vi "obj_DataLog Tag Hash.vi"(0 "method":T1=enum."index tag", 7 "tag in":string, 9 "tag index in":i32=-1, 11 "error in (no error)":errorcluster) -> (6 "#tags":i32, 8 "tag out":string, 10 "tag index out":i32, 15 "error out":errorcluster)   [LabVIEW 2012]
doc: "Efficiently associates the names of the tags in the live database with their indices. A tag index is required to access tag-specific data inside data structures set up for the live database. Only the {index tag}, {lookup}, and {#tags} methods are meant for public use. The {index tag} method retrieves the tag's name given a tag index. The {lookup} method retrieves the tag's index given a tag name. The {#tags} method returns the number of tags in the live database.\n\nBy storing the tag indices in a hash table, a lookup of a tag's index via its name becomes an O(1) operation (the execution time is independent of the number of tags). In this way, the amount of work during repeated run-time operations is reduced by proper preparation during the once-only initialization.\n\nNOTE: the subVIs for accessing the live database mostly accept both tag indices and tag names. In the latter case, they use this object to {lookup} the tag index."
uses:
  typedefs/t_DataLog Tag Hash Methods.ctl
  subvis/private/glb_DataLog Runtime Parameterisation.vi
  subvis/private/glb_DataLog MCVD.vi
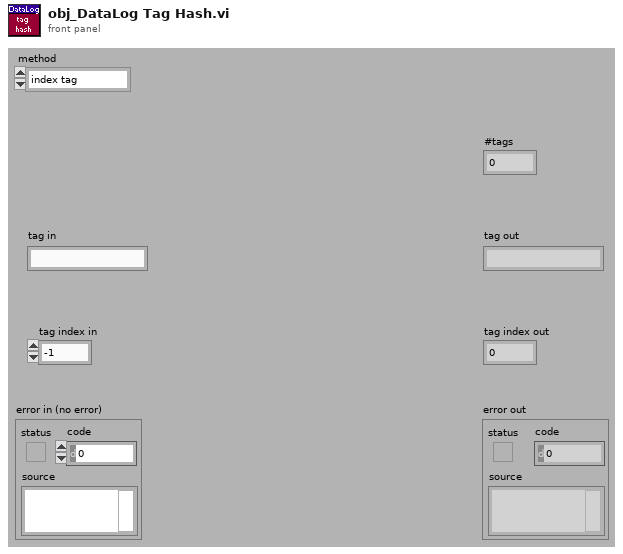
[diagram p1: front panel]
types:
  T1 = typedef "t_DataLog Tag Hash Methods.ctl" = enum16{"initialize", "add tag", "index tag", "lookup", "#tags", "cleanup", "write recovery", "read recovery", "delete recovery"}
  T2 = enum16{"deny read/write", "deny write-only", "deny none"}
  T3 = enum16{"read/write", "read-only", "write-only", "write-only (truncate)"}
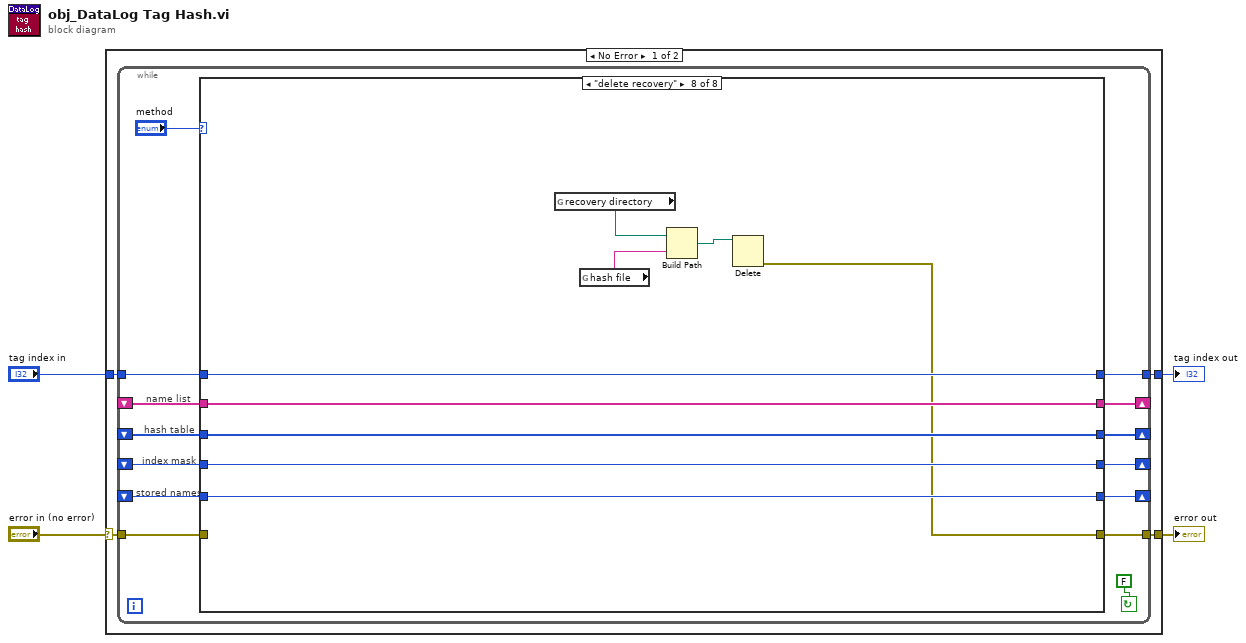
[diagram p0: block diagram]
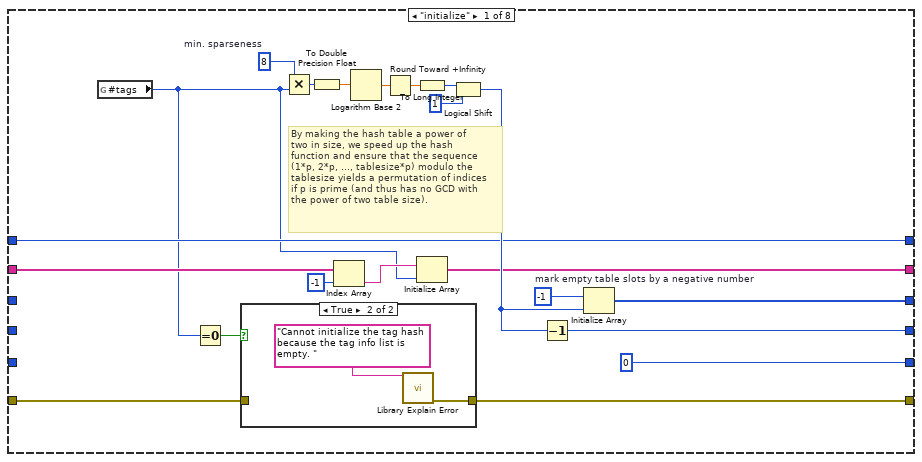
[diagram p2: hidden frame]
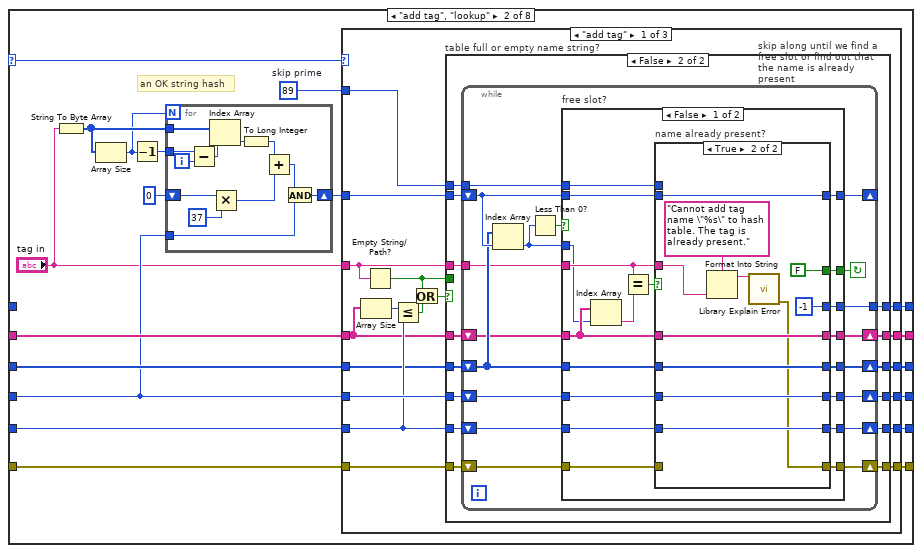
[diagram p4: hidden frame]
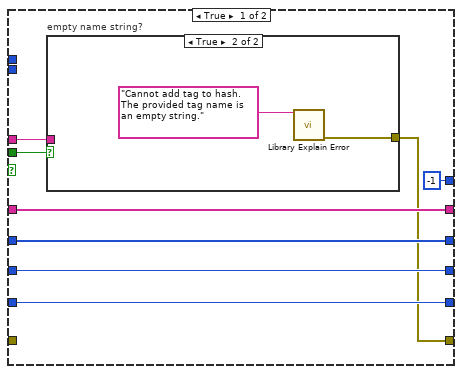
[diagram p5: hidden frame]
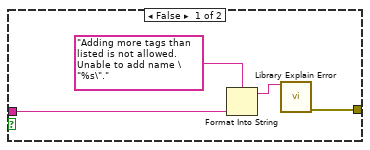
[diagram p6: hidden frame]
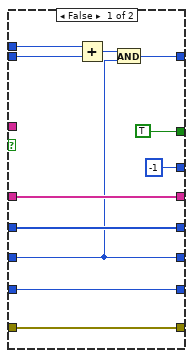
[diagram p7: hidden frame]
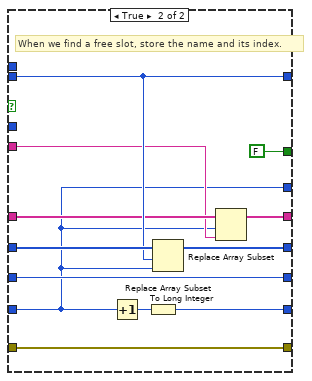
[diagram p8: hidden frame]
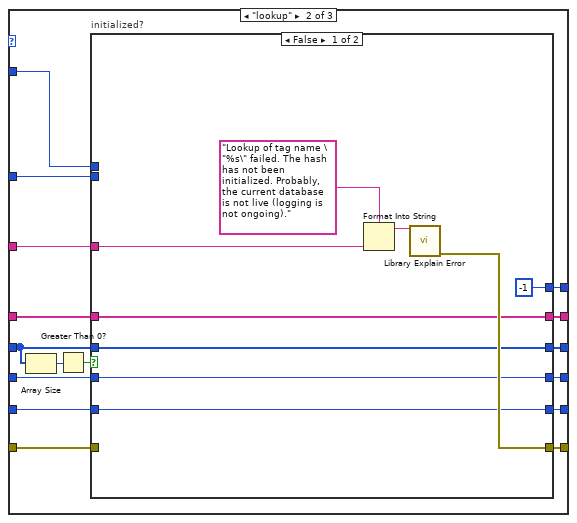
[diagram p9: hidden frame]
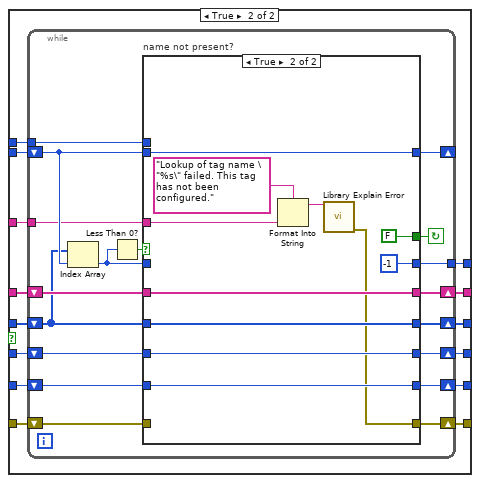
[diagram p10: hidden frame]
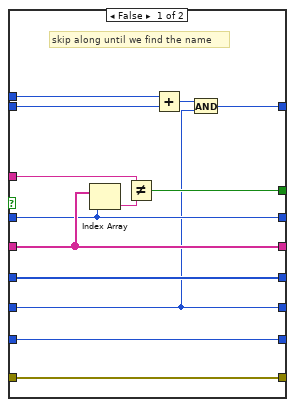
[diagram p11: hidden frame]
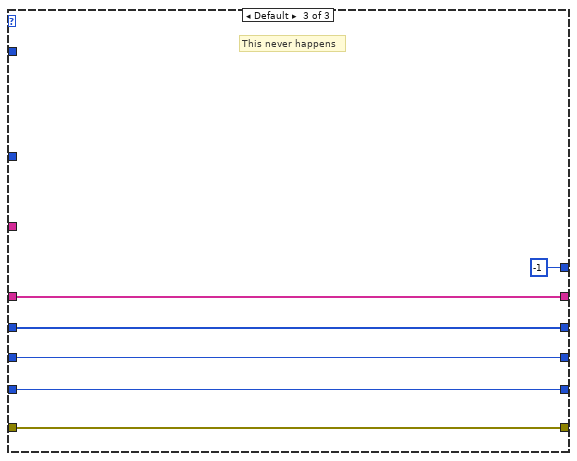
[diagram p12: hidden frame]
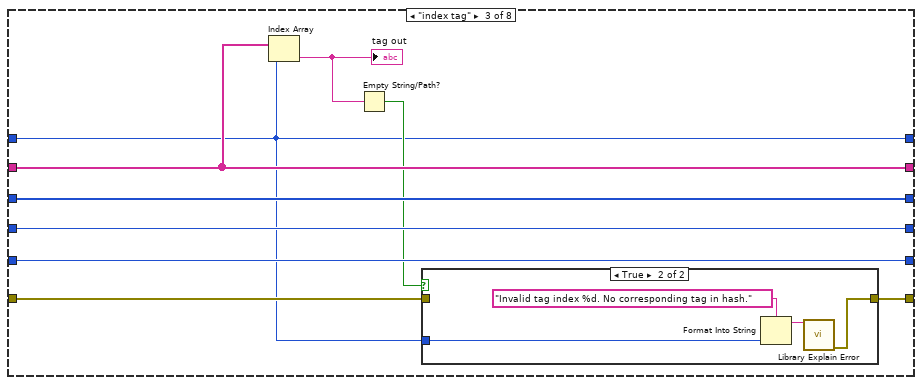
[diagram p13: hidden frame]
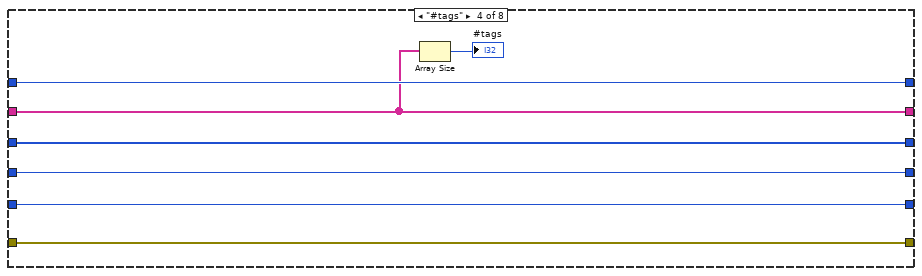
[diagram p15: hidden frame]
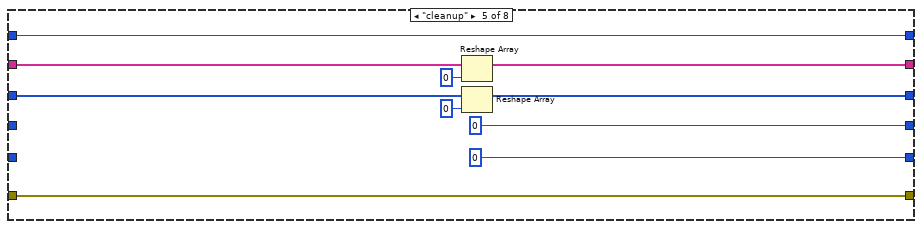
[diagram p16: hidden frame]
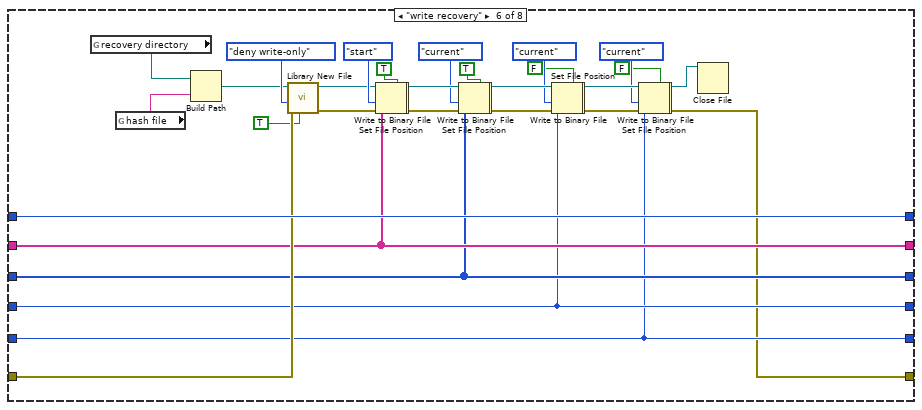
[diagram p17: hidden frame]
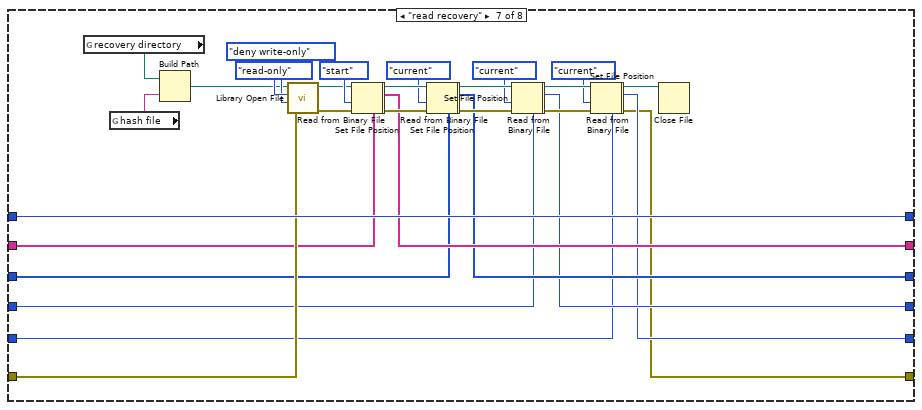
[diagram p18: hidden frame]
diagram:
  n1 = case shown="No Error" "error in (no error)" {
    selector: "error in (no error)" -> [w8 w397]
    tunnel: [w7 w397] -> w3
    tunnel: "tag index in" -> [w6 w396]
    tunnel: [w5 w396] -> w1
    frame No Error {
      n2 = while {
        shift-right: [w21] -> _
        shift-left: _ -> [w16]
        tunnel: w8 -> [w14]
        tunnel: [w20] -> w7
        shift-right: [w19] -> _
        shift-left: _ -> [w17]
        shift-right: [w18] -> _
        shift-left: _ -> [w15]
        tunnel: w6 -> [w12]
        tunnel: [w11] -> w5
        shift-right: [w9] -> _
        shift-left: _ -> [w10]
        stop <- FALSE continue-if-true
        # "stored names"
        # "index mask"
        # "name list"
        # "hash table"
        n3 = case shown="\"delete recovery\"" "method" {
          selector: "method" -> [_ w52 _ _ _ _ _ _]
          tunnel: w16 -> [_ w57 w289 w301 w306 w332 w366 w391]
          tunnel: [w31 w58 w289 w301 w305 w332 w367 w391] -> w21
          tunnel: w14 -> [w24 w53 w284 w299 w312 w334 w370 _]
          tunnel: [w26 w54 w283 w299 w312 w324 w359 w388] -> w20
          tunnel: w17 -> [w28 w60 w287 w297 w308 w333 w369 w392]
          tunnel: [w27 w59 w287 w297 w307 w333 w368 w392] -> w19
          tunnel: [w34 w55 w290 w302 0 w331 w365 w390] -> w18
          tunnel: w15 -> [_ w56 w290 w302 _ w331 w364 w390]
          tunnel: w12 -> [w32 _ w282 w298 w310 w349 w386 w395]
          tunnel: [w32 w61 w282 w298 w310 w349 w386 w395] -> w11
          tunnel: w10 -> [_ w49 w288 w300 _ w330 w362 w389]
          tunnel: [0 w48 w288 w300 0 w330 w363 w389] -> w9
          frame "initialize" {
            w36 = -1  # mark empty table slots by a negative number
            w37 = 8  # min. sparseness
            # "By making the hash table a power of\ntwo in size, we speed up the hash\nfunction and ensure that the sequence\n(1*p, 2*p, ..., tablesize*p) modulo the\ntablesize yields a permutation of indices\nif p is prime (and thus has no GCD with\nthe power of two table size)."
            n4 = global read "glb_DataLog Runtime Parameterisation.vi" "#tags"() -> (w23:i32)
            n5 = Equal To 0?(x=w23) -> (x = 0?=w25:bool)
            n6 = case shown="True" w25 {
              tunnel: [w44 w46] -> w26
              tunnel: w24 -> [w44 _]
              frame False {
              }
              frame True {
                n7 = call "Library Explain Error.vi"("explanation prefix (none)"="Cannot initialize the tag hash because the tag info list is empty. " ("explanation")) -> ("explained error"=w46:errorcluster)  [unwired: 14 in]
              }
            }
            n8 = Multiply(x=w37, y=w23) -> (x*y=w38:i32)
            n9 = To Double Precision Float(number=w38) -> (double precision float=w43:dbl)
            n10 = Index Array(array=w28, index=-1) -> (element=w29:string)
            n11 = Logarithm Base 2(1:w43) -> (0:w42:dbl)
            n12 = Round Toward +Infinity(x=w42) -> (ceil(x): smallest int >= x=w41:dbl)
            n13 = To Long Integer(number=w41) -> (32bit integer=w40:i32)
            n14 = Initialize Array(w29, w23) -> (w27:string[])
            n15 = Logical Shift(y=w40, x=1) -> (x << y=w35:i32)
            n16 = Decrement(x=w35) -> (x-1=w34:i32)
            n17 = Initialize Array(w36, w35) -> (w31:i32[])
          }
          frame "add tag", "lookup" {
            w47 = 89  # skip prime
            # "an OK string hash"
            n18 = String To Byte Array(string="tag in") -> (unsigned byte array=w64:u8[])
            n19 = Array Size(array=w64) -> (size(s)=w62:i32)
            n20 = Decrement(x=w62) -> (x-1=w63:i32)
            n21 = for {
              N: w62 -> [_]
              shift-right: [w275] -> w50
              shift-left: 0 -> [w276]
              tunnel: w64 -> [w279]
              tunnel: w63 -> [w281]
              tunnel: w56 -> [w274]
              i -> [w280]
              n22 = Subtract(x=w281, y=w280) -> (x-y=w278:i32)
              n23 = Index Array(array=w279, index=w278) -> (element=w273:u8)
              n24 = Multiply(x=w276, y=37 ("x")) -> (x*y=w272:i32)
              n25 = To Long Integer(number=w273) -> (32bit integer=w271:i32)
              n26 = Add(x=w271, y=w272) -> (x+y=w270:i32)
              n27 = And(x=w270, y=w274) -> (x .and. y?=w275:i32)
            }
            n28 = case shown="\"add tag\"" w52 {
              tunnel: [w75 w187 -1] -> w61
              tunnel: w60 -> [w67 w190 w269]
              tunnel: [w76 w194 w269] -> w59
              tunnel: w57 -> [w69 w186 w268]
              tunnel: [w81 w195 w268] -> w58
              tunnel: [w79 w196 w267] -> w55
              tunnel: w56 -> [w83 w191 w267]
              tunnel: w53 -> [w77 w193 w266]
              tunnel: [w78 w198 w266] -> w54
              tunnel: "tag in" -> [w71 w188 _]
              tunnel: w50 -> [w82 w189 _]
              tunnel: w49 -> [w74 w192 w264]
              tunnel: [w80 w197 w264] -> w48
              tunnel: w47 -> [w66 w183 _]
              frame "add tag" {
                n29 = Array Size(array=w67) -> (size(s)=w68:i32)
                n30 = Empty String/Path?(string/path=w71) -> (empty?=w70:bool)
                n31 = Less Or Equal?(x=w68, y=w74) -> (x <= y?=w73:bool)
                n32 = Or(x=w70, y=w73) -> (x .or. y?=w72:bool)
                n33 = case "table full or empty name string?" shown="False" w72 {
                  tunnel: w83 -> [w89 w105]
                  tunnel: w82 -> [_ w111]
                  tunnel: w69 -> [w90 w104]
                  tunnel: w74 -> [w88 w101]
                  tunnel: [w90 w110] -> w81
                  tunnel: [w88 w107] -> w80
                  tunnel: [w89 w106] -> w79
                  tunnel: [w84 w108] -> w78
                  tunnel: w77 -> [_ w109]
                  tunnel: w67 -> [w91 w103]
                  tunnel: [w91 w102] -> w76
                  tunnel: [-1 w100] -> w75
                  tunnel: w71 -> [w85 w99]
                  tunnel: w70 -> [w86 _]
                  tunnel: w66 -> [_ w98]
                  frame True {
                    n34 = case "empty name string?" shown="True" w86 {
                      tunnel: w85 -> [w95 _]
                      tunnel: [w92 w96] -> w84
                      frame False {
                        n35 = Format Into String(format string="Adding more tags than listed is not allowed. Unable to add name \"%s\".", w95) -> (resulting string=w93:string)  [unwired: 2 in, 1 out]
                        n36 = call "Library Explain Error.vi"("explanation prefix (none)"=w93) -> ("explained error"=w92:errorcluster)  [unwired: 14 in]
                      }
                      frame True {
                        n37 = call "Library Explain Error.vi"("explanation prefix (none)"="Cannot add tag to hash. The provided tag name is an empty string." ("explanation")) -> ("explained error"=w96:errorcluster)  [unwired: 14 in]
                      }
                    }
                  }
                  frame False {
                    n38 = while "skip along until we find a free slot or find out that the name is already present" {
                      shift-right: [w128] -> _
                      shift-left: w111 -> [w129]
                      shift-right: [w126] -> w110
                      shift-left: w104 -> [w127]
                      shift-right: [w123] -> w108
                      shift-left: w109 -> [w124]
                      shift-right: [w121] -> w107
                      shift-left: w101 -> [w122]
                      shift-right: [w119] -> w106
                      shift-left: w105 -> [w120]
                      shift-right: [w114] -> w102
                      shift-left: w103 -> [w115]
                      tunnel: [w118] -> w100
                      tunnel: w99 -> [w113]
                      tunnel: w98 -> [w112]
                      stop <- w125 continue-if-true
                      n39 = Index Array(array=w127, index=w129) -> (element=w117:i32)
                      n40 = Less Than 0?(x=w117) -> (x < 0?=w116:bool)
                      n41 = case "free slot?" shown="False" w116 {
                        tunnel: w129 -> [w144 w180]
                        tunnel: [w145 w180] -> w128
                        tunnel: w127 -> [w148 w182]
                        tunnel: [w147 w176] -> w126
                        tunnel: w117 -> [w131 _]
                        tunnel: [w146 FALSE] -> w125
                        tunnel: [w141 w179] -> w123
                        tunnel: w124 -> [w142 w179]
                        tunnel: w122 -> [w140 w172]
                        tunnel: [w139 w173] -> w121
                        tunnel: w120 -> [w138 w178]
                        tunnel: [w137 w178] -> w119
                        tunnel: [w133 w172] -> w118
                        tunnel: w115 -> [w136 w175]
                        tunnel: [w135 w171] -> w114
                        tunnel: w113 -> [w132 w174]
                        tunnel: w112 -> [w130 _]
                        frame False {
                          n42 = Index Array(array=w136, index=w131) -> (element=w143:string)
                          n43 = Equal?(x=w132, y=w143) -> (x = y?=w134:bool)
                          n44 = case "name already present?" shown="True" w134 {
                            tunnel: w148 -> [w152 w166]
                            tunnel: [w152 w166] -> w147
                            tunnel: [TRUE FALSE] -> w146
                            tunnel: [w158 w165] -> w145
                            tunnel: w140 -> [w151 w167]
                            tunnel: w144 -> [w157 w165]
                            tunnel: w142 -> [w155 _]
                            tunnel: [w155 w161] -> w141
                            tunnel: [w151 w167] -> w139
                            tunnel: w138 -> [w150 w169]
                            tunnel: [w150 w169] -> w137
                            tunnel: w136 -> [w154 w168]
                            tunnel: [w154 w168] -> w135
                            tunnel: [-1 -1] -> w133
                            tunnel: w132 -> [_ w162]
                            tunnel: w130 -> [w149 _]
                            frame False {
                              n45 = Add(x=w149, y=w157) -> (x+y=w156:i32)
                              n46 = And(x=w156, y=w150) -> (x .and. y?=w158:i32)
                            }
                            frame True {
                              n47 = Format Into String(format string="Cannot add tag name \"%s\" to hash table. The tag is already present.", w162) -> (resulting string=w160:string)  [unwired: 2 in, 1 out]
                              n48 = call "Library Explain Error.vi"("explanation prefix (none)"=w160) -> ("explained error"=w161:errorcluster)  [unwired: 14 in]
                            }
                          }
                        }
                        frame True {
                          # "When we find a free slot, store the name and its index."
                          n49 = Increment(x=w172) -> (x+1=w177:i32)
                          n50 = To Long Integer(number=w177) -> (32bit integer=w173:i32)
                          n51 = Replace Array Subset(array=w182, new element=w172, index=w180) -> (w176:i32[])
                          n52 = Replace Array Subset(array=w175, new element=w174, index=w172) -> (w171:string[])
                        }
                      }
                    }
                  }
                }
              }
              frame "lookup" {
                n53 = Array Size(array=w186) -> (size(s)=w185:i32)
                n54 = Greater Than 0?(x=w185) -> (x > 0?=w184:bool)
                n55 = case "initialized?" shown="False" w184 {
                  tunnel: [w205 w221] -> w198
                  tunnel: [w200 w220] -> w197
                  tunnel: [w201 w219] -> w196
                  tunnel: [w202 w218] -> w195
                  tunnel: [w203 w217] -> w194
                  tunnel: w193 -> [_ w216]
                  tunnel: w192 -> [w200 w215]
                  tunnel: w191 -> [w201 w214]
                  tunnel: w186 -> [w202 w213]
                  tunnel: w190 -> [w203 w212]
                  tunnel: w189 -> [_ w211]
                  tunnel: w188 -> [w204 w210]
                  tunnel: [-1 w209] -> w187
                  tunnel: w183 -> [_ w208]
                  frame False {
                    n56 = Format Into String(format string="Lookup of tag name \"%s\" failed. The hash has not been initialized. Probably, the current database is not live (logging is not ongoing).", w204) -> (resulting string=w206:string)  [unwired: 2 in, 1 out]
                    n57 = call "Library Explain Error.vi"("explanation prefix (none)"=w206) -> ("explained error"=w205:errorcluster)  [unwired: 14 in]
                  }
                  frame True {
                    n58 = while {
                      shift-right: [w236] -> w221
                      shift-left: w216 -> [w237]
                      shift-right: [w234] -> w220
                      shift-left: w215 -> [w235]
                      shift-right: [w232] -> w219
                      shift-left: w214 -> [w233]
                      shift-right: [w231] -> w218
                      shift-left: w213 -> [w224]
                      shift-right: [w229] -> w217
                      shift-left: w212 -> [w230]
                      shift-right: [w239] -> _
                      shift-left: w211 -> [w238]
                      tunnel: w210 -> [w228]
                      tunnel: [w226] -> w209
                      tunnel: w208 -> [w222]
                      stop <- w227 continue-if-true
                      n59 = Index Array(array=w224, index=w238) -> (element=w225:i32)
                      n60 = Less Than 0?(x=w225) -> (x < 0?=w223:bool)
                      n61 = case "name not present?" shown="True" w223 {
                        tunnel: [w252 w254] -> w239
                        tunnel: w233 -> [w241 w262]
                        tunnel: w238 -> [w251 w254]
                        tunnel: w237 -> [w244 _]
                        tunnel: [w244 w255] -> w236
                        tunnel: w235 -> [w242 w263]
                        tunnel: [w242 w263] -> w234
                        tunnel: [w241 w262] -> w232
                        tunnel: w224 -> [w250 w261]
                        tunnel: [w250 w261] -> w231
                        tunnel: w230 -> [w249 w260]
                        tunnel: [w249 w260] -> w229
                        tunnel: w228 -> [w247 w257]
                        tunnel: [w243 FALSE] -> w227
                        tunnel: [w246 -1] -> w226
                        tunnel: w225 -> [w246 _]
                        tunnel: w222 -> [w240 _]
                        frame False {
                          # "skip along until we find the name"
                          n62 = Index Array(array=w249, index=w246) -> (element=w248:string)
                          n63 = Not Equal?(x=w247, y=w248) -> (x != y?=w243:bool)
                          n64 = Add(x=w240, y=w251) -> (x+y=w245:i32)
                          n65 = And(x=w245, y=w241) -> (x .and. y?=w252:i32)
                        }
                        frame True {
                          n66 = Format Into String(format string="Lookup of tag name \"%s\" failed. This tag has not been configured.", w257) -> (resulting string=w258:string)  [unwired: 2 in, 1 out]
                          n67 = call "Library Explain Error.vi"("explanation prefix (none)"=w258) -> ("explained error"=w255:errorcluster)  [unwired: 14 in]
                        }
                      }
                    }
                  }
                }
              }
              frame Default {
                # "This never happens"
              }
            }
          }
          frame "index tag" {
            n68 = Index Array(array=w287, index=w282) -> (element=w286:string)
            "tag out" <- w286
            n69 = Empty String/Path?(string/path=w286) -> (empty?=w285:bool)
            n70 = case shown="True" w285 {
              tunnel: w284 -> [w291 _]
              tunnel: [w291 w292] -> w283
              tunnel: w282 -> [_ w294]
              frame False {
              }
              frame True {
                n71 = Format Into String(format string="Invalid tag index %d. No corresponding tag in hash.", w294) -> (resulting string=w295:string)  [unwired: 2 in, 1 out]
                n72 = call "Library Explain Error.vi"("explanation prefix (none)"=w295) -> ("explained error"=w292:errorcluster)  [unwired: 14 in]
              }
            }
          }
          frame "#tags" {
            n73 = Array Size(array=w297) -> (size(s)=→"#tags":i32)
          }
          frame "cleanup" {
            n74 = Reshape Array(w308, 0 ("dimension size")) -> (w307:string[])
            n75 = Reshape Array(w306, 0 ("dimension size")) -> (w305:i32[])
          }
          frame "write recovery" {
            n76 = global read "glb_DataLog Runtime Parameterisation.vi" "recovery directory"() -> (w323:path)
            n77 = global read "glb_DataLog MCVD.vi" "hash file"() -> (w327:string)
            n78 = Build Path(base path=w323, name or relative path=w327) -> (appended path=w328:path)
            n79 = call "Library New File.vi"("overwrite (F)"=TRUE, "error in (no error)"=w334, "deny mode (deny none)"=T2."deny write-only" ("deny mode (2)"), "file path"=w328) -> ("error out"=w346:errorcluster, "refnum"=w345:refnum<file>)  [unwired: 6 in]
            n80 = Set File Position(refnum=w345, from (0:start)=enum16{"start", "end", "current"}."start" ("pos mode (0:2)"), error in=w346) -> (refnum out=w314:refnum<file>, error out=w313:errorcluster)  [unwired: 1 in]
            n81 = Write to Binary File(file (use dialog)=w314, data=w333, error in=w313, 5:TRUE ("header (F)")) -> (refnum out=w339:refnum<file>, error out=w340:errorcluster)  [unwired: 2 in, 1 out]
            n82 = Set File Position(refnum=w339, from (0:start)=enum16{"start", "end", "current"}."current" ("pos mode (0:2)"), error in=w340) -> (refnum out=w316:refnum<file>, error out=w315:errorcluster)  [unwired: 1 in]
            n83 = Write to Binary File(file (use dialog)=w316, data=w332, error in=w315, 5:TRUE ("header (F)")) -> (refnum out=w341:refnum<file>, error out=w342:errorcluster)  [unwired: 2 in, 1 out]
            n84 = Set File Position(refnum=w341, from (0:start)=enum16{"start", "end", "current"}."current" ("pos mode (0:2)"), error in=w342) -> (refnum out=w319:refnum<file>, error out=w318:errorcluster)  [unwired: 1 in]
            n85 = Write to Binary File(file (use dialog)=w319, data=w331, error in=w318, 5:FALSE ("prepend array or string size? (T)")) -> (refnum out=w343:refnum<file>, error out=w344:errorcluster)  [unwired: 2 in, 1 out]
            n86 = Set File Position(refnum=w343, from (0:start)=enum16{"start", "end", "current"}."current" ("pos mode (0:2)"), error in=w344) -> (refnum out=w322:refnum<file>, error out=w321:errorcluster)  [unwired: 1 in]
            n87 = Write to Binary File(file (use dialog)=w322, data=w330, error in=w321, 5:FALSE ("prepend array or string size? (T)")) -> (refnum out=w338:refnum<file>, error out=w324:errorcluster)  [unwired: 2 in, 1 out]
            n88 = Close File(refnum=w338) -> ()  [unwired: 1 in, 2 out]
          }
          frame "read recovery" {
            n89 = global read "glb_DataLog Runtime Parameterisation.vi" "recovery directory"() -> (w358:path)
            n90 = global read "glb_DataLog MCVD.vi" "hash file"() -> (w361:string)
            n91 = Build Path(base path=w358, name or relative path=w361) -> (appended path=w360:path)
            n92 = call "Library Open File.vi"("error in (no error)"=w370, "deny mode (deny none)"=T2."deny write-only" ("deny mode (2)"), "open mode (read/write)"=T3."read-only" ("open mode (0)"), "file path"=w360) -> ("error out"=w382:errorcluster, "refnum"=w381:refnum<file>)  [unwired: 2 in]
            n93 = Set File Position(refnum=w381, from (0:start)=enum16{"start", "end", "current"}."start" ("pos mode (0:2)"), error in=w382) -> (refnum out=w351:refnum<file>, error out=w350:errorcluster)  [unwired: 1 in]
            n94 = Read from Binary File(5:w369, 8:w350, 11:w351) -> (0:w376:errorcluster, 2:w368:string[], 3:w375:refnum<file>)  [unwired: 3 in, 1 out]
            n95 = Set File Position(refnum=w375, from (0:start)=enum16{"start", "end", "current"}."current" ("pos mode (0:2)"), error in=w376) -> (refnum out=w353:refnum<file>, error out=w352:errorcluster)  [unwired: 1 in]
            n96 = Read from Binary File(5:w366, 8:w352, 11:w353) -> (0:w378:errorcluster, 2:w367:i32[], 3:w377:refnum<file>)  [unwired: 3 in, 1 out]
            n97 = Set File Position(refnum=w377, from (0:start)=enum16{"start", "end", "current"}."current" ("pos mode (0:2)"), error in=w378) -> (refnum out=w355:refnum<file>, error out=w354:errorcluster)  [unwired: 1 in]
            n98 = Read from Binary File(5:w364, 8:w354, 11:w355) -> (0:w380:errorcluster, 2:w365:i32, 3:w379:refnum<file>)  [unwired: 3 in, 1 out]
            n99 = Set File Position(refnum=w379, from (0:start)=enum16{"start", "end", "current"}."current" ("pos mode (0:2)"), error in=w380) -> (refnum out=w357:refnum<file>, error out=w356:errorcluster)  [unwired: 1 in]
            n100 = Read from Binary File(5:w362, 8:w356, 11:w357) -> (0:w359:errorcluster, 2:w363:i32, 3:w374:refnum<file>)  [unwired: 3 in, 1 out]
            n101 = Close File(refnum=w374) -> ()  [unwired: 1 in, 2 out]
          }
          frame "delete recovery" {
            n102 = global read "glb_DataLog Runtime Parameterisation.vi" "recovery directory"() -> (w387:path)
            n103 = global read "glb_DataLog MCVD.vi" "hash file"() -> (w394:string)
            n104 = Build Path(base path=w387, name or relative path=w394) -> (appended path=w393:path)
            n105 = Delete(path (use dialog)=w393) -> (error out=w388:errorcluster)  [unwired: 4 in, 2 out]
          }
        }
      }
    }
    frame Error {
    }
  }
  "error out" <- w3
  "tag index out" <- w1
